vi "Create.vi"(8 "error in (no error)":errorcluster, 10 "Variables":map{string, dbl}(c390)) -> (0 "error out":errorcluster, 3 "Variables out":refnum<class "Variables.lvclass">)   [LabVIEW 2020, in "VolatusSeq.lvlib" / "Variables.lvclass"]
uses:
  Variables.lvclass
  Variables.lvclass/Variables.ctl
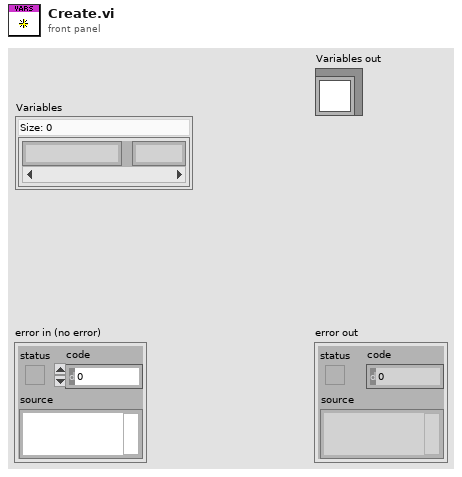
[diagram p1: front panel]
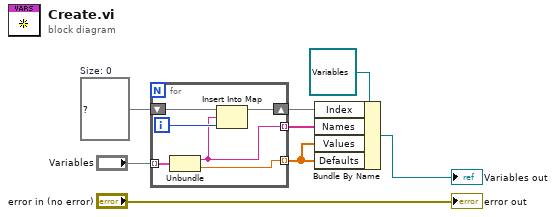
[diagram p0: block diagram]
diagram:
  w4 = map{string, i32} {}  # Size: 0
  n1 = for {
    tunnel: "Variables" -> [w12] mode=indexing
    shift-right: [w11] -> w3
    shift-left: w4 -> [w14]
    tunnel: [w10] -> w2 mode=indexing
    tunnel: [w9] -> w1 mode=indexing
    i -> [w13]
    n2 = Unbundle(w12) -> ("Name"=w10:string, "Value"=w9:dbl)
    n3 = Insert Into Map(map in=w14, key=w10, value=w13) -> (map out=w11:map{string, i32})  [unwired: 2 out]
  }
  n4 = Bundle By Name(cluster=refnum<class "Variables.lvclass"> refnum ("Variables in"), "Index"=w3, "Names"=w2, "Values"=w1, "Defaults"=w1) -> (→"Variables out":refnum<class "Variables.lvclass">)
  "error out" <- "error in (no error)"
